vi "Sec till next shot.vi"(8 "error in (no error)":errorcluster, 11 "BME_DG_Chnl in":refnum<class "BME_DG_Chnl.lvclass">) -> (0 "error out":errorcluster, 2 "sec till next shot":dbl, 3 "BME_DG_Chnl out":refnum<class "BME_DG_Chnl.lvclass">)   [LabVIEW 2009, in "POLARIS BME DG.lvlib" / "BME_DG_Chnl.lvclass"]
uses:
  BME_DG_Chnl.lvclass
  BME_DG_Chnl.lvclass/BME_DG_Chnl.ctl
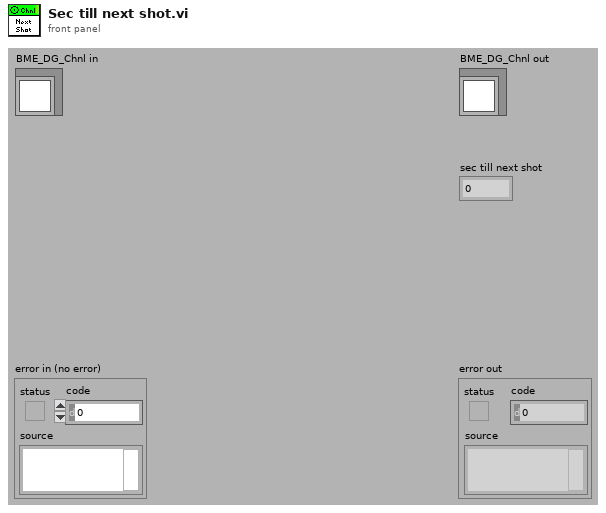
[diagram p1: front panel]
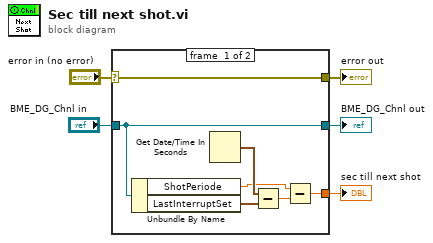
[diagram p0: block diagram]
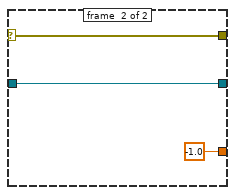
[diagram p2: hidden frame]
diagram:
  n1 = case shown="No Error" "error in (no error)" {
    selector: "error in (no error)" -> [w12 w15]
    tunnel: [w12 w15] -> w4
    tunnel: [w11 w14] -> w2
    tunnel: "BME_DG_Chnl in" -> [w11 w14]
    tunnel: [w6 -1.0] -> w1
    frame #0 {
      n2 = Unbundle By Name(w11) -> ("ShotPeriode"=w8:dbl, "LastInterruptSet"=w10:timestamp)
      n3 = Get Date/Time In Seconds() -> (seconds since 1Jan1904=w9:timestamp)
      n4 = Subtract(x=w9, y=w10) -> (x-y=w7:dbl)
      n5 = Subtract(x=w8, y=w7) -> (x-y=w6:dbl)
    }
    frame #1 {
    }
  }
  "error out" <- w4
  "BME_DG_Chnl out" <- w2
  "sec till next shot" <- w1
